vi "GetTimeout.vi"(8 "error in (no error)":errorcluster, 11 "ScopeBase in":refnum<class "ScopeBase.lvclass">) -> (0 "error out":errorcluster, 1 "Time left":i32, 3 "ScopeBase out":refnum<class "ScopeBase.lvclass">)   [LabVIEW 2013, in "ScopeBase.lvclass"]
uses:
  ScopeBase.lvclass
  ScopeBase.lvclass/ScopeBase.ctl
  Utilities/Ticker/Ticker.lvclass
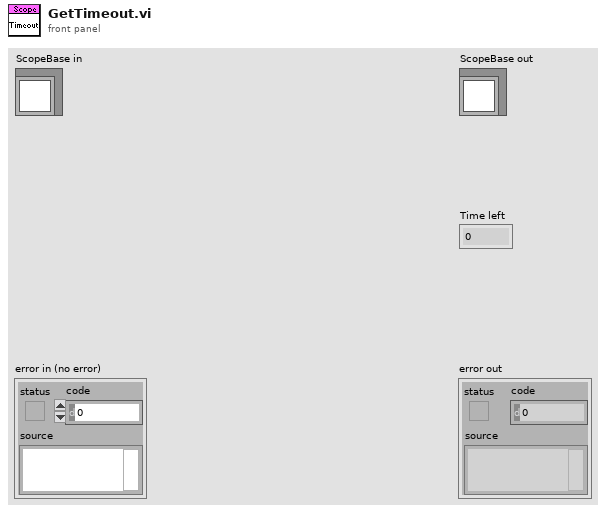
[diagram p1: front panel]
types:
  T1 = typedef "ScopeMode.ctl" = enum16{"Stopped", "Single", "Running", "Continuous"}
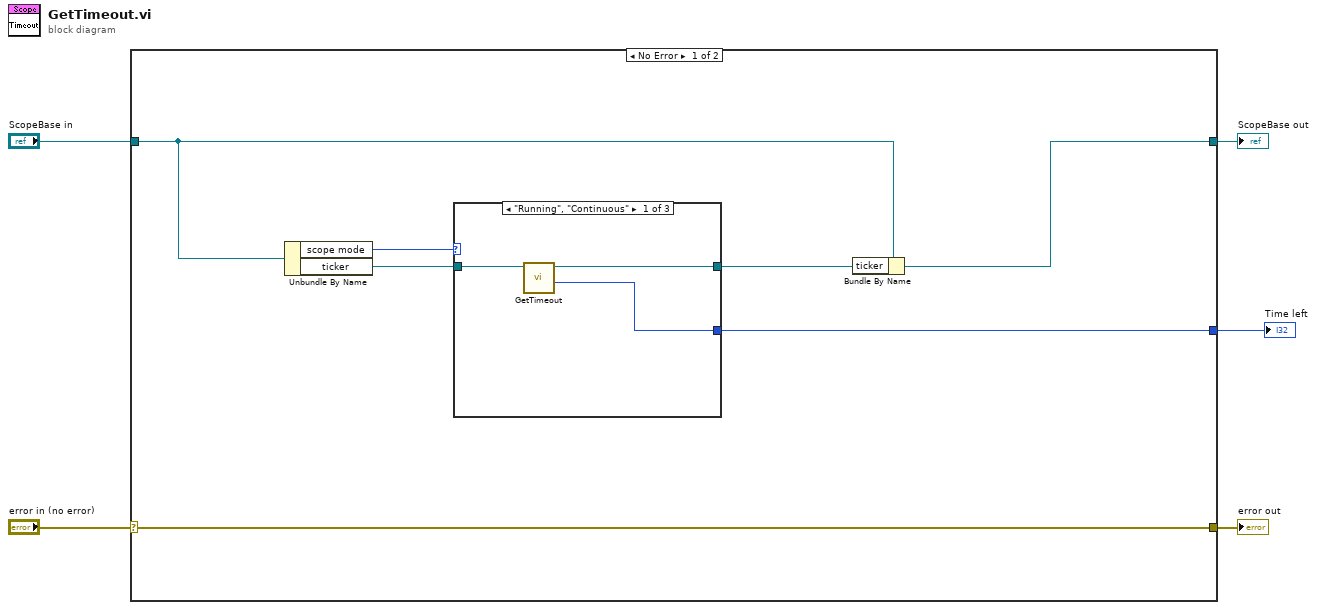
[diagram p0: block diagram]
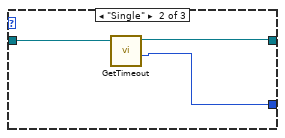
[diagram p2: hidden frame]
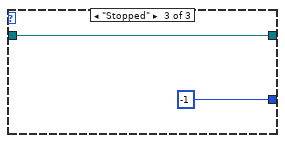
[diagram p3: hidden frame]
diagram:
  n1 = case shown="No Error" "error in (no error)" {
    selector: "error in (no error)" -> [w12 w22]
    tunnel: [w12 w22] -> w4
    tunnel: [w7 w21] -> w2
    tunnel: "ScopeBase in" -> [w8 w21]
    tunnel: [w6 _] -> w1
    frame No Error {
      n2 = Unbundle By Name(w8) -> ("scope mode"=w11:T1, "ticker"=w10:refnum<class "Ticker.lvclass">)
      n3 = case shown="\"Running\", \"Continuous\"" w11 {
        tunnel: w10 -> [w15 w18 w19]
        tunnel: [w14 w16 -1 ("Time left")] -> w6
        tunnel: [w13 w17 w19] -> w9
        frame "Running", "Continuous" {
          n4 = call "GetTimeout.vi"("Ticker In"=w15) -> ("Time left"=w14:i32, "Ticker Out"=w13:refnum<class "Ticker.lvclass">)  [unwired: 7 in, 2 out]
        }
        frame "Single" {
          n5 = call "GetTimeout.vi"("Ticker In"=w18) -> ("Time left"=w16:i32, "Ticker Out"=w17:refnum<class "Ticker.lvclass">)  [unwired: 7 in, 2 out]
        }
        frame "Stopped" {
        }
      }
      n6 = Bundle By Name(cluster=w8, "ticker"=w9) -> (w7:refnum<class "ScopeBase.lvclass">)
    }
    frame Error {
    }
  }
  "error out" <- w4
  "ScopeBase out" <- w2
  "Time left" <- w1
